vi "Open.vi"(7 "Allow multiple opens?":bool, 8 "error in (no error)":errorcluster, 10 "Channel Names":tag[](array[tag])) -> (0 "error out":errorcluster, 3 "AudioIn (N Samples) Ref Out":T1)   [LabVIEW 2021, in "AudioIn Block.lvlib"]
doc: "Opens a reference to audio input block read channels. You must open a reference before you read values from the audio input block read channels."
uses:
  <vilib>/myRIO/Instrument Drivers/Onboard IO/AudioIn Block/AudioIn Block.lvlib
  <vilib>/myRIO/Instrument Drivers/Onboard IO/AudioIn Block/typedefs/AudioIn Block Reference.ctl
  <vilib>/myRIO/Common/Instrument Driver Framework/Utilities/typedefs/myRIO Generic Hardware Reference.ctl
  <vilib>/myRIO/Common/Instrument Driver Framework/Utilities/typedefs/Hardware Version Enum.ctl
  <vilib>/myRIO/Common/Instrument Driver Framework/Utilities/typedefs/myRIO v1.0 Reference.ctl
  <vilib>/myRIO/Common/Instrument Driver Framework/Utilities/typedefs/Generic FPGA Reference.ctl
  <vilib>/myRIO/Common/Instrument Driver Framework/myRIO v1.0/AudioIn Block/typedefs/AudioIn Block Channels List.ctl
  <vilib>/myRIO/Common/Instrument Driver Framework/myRIO v1.0/AudioIn Block/typedefs/AudioIn Block Channels Enum.ctl
  <vilib>/myRIO/Common/Instrument Driver Framework/Utilities/typedefs/Analog Scaling Constants.ctl
  <vilib>/userdefined/High Color/nirio_resource_hc.ctl
panel:
  # "AudioIn (N Samples) Open"
  # "Opens a reference to the myRIO hardware and configures the AudioIn (N Samples) Reference with channels to be read"
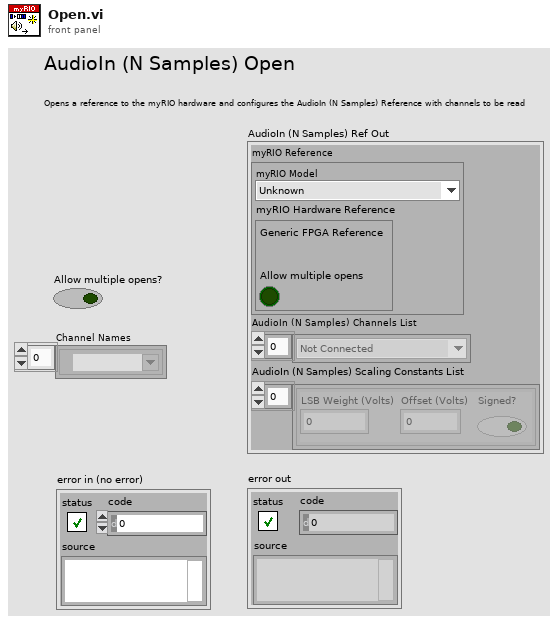
[diagram p1: front panel]
types:
  T1 = typedef "AudioIn Block.lvlib/AudioIn Block Reference.ctl" = cluster{"myRIO Reference":T2, "AudioIn (N Samples) Channels List":T6, "AudioIn (N Samples) Scaling Constants List":T8[]}
  T2 = typedef "myRIO Generic Hardware Reference.ctl" = cluster{"myRIO Model":T3, "myRIO Hardware Reference":T4}
  T3 = typedef "Hardware Version Enum.ctl" = enum16{"Unknown", "myRIO-1900", "myRIO-1950", "roboRIO", "NI ELVIS RIO CM", "ELVIS III"}
  T4 = typedef "myRIO v1.0 Reference.ctl" = cluster{"Generic FPGA Reference":T5, "Allow multiple opens":bool}
  T5 = typedef "Generic FPGA Reference.ctl" = refnum<k20>
  T6 = typedef "AudioIn Block Channels List.ctl" = T7[]
  T7 = typedef "AudioIn Block Channels Enum.ctl" = enum16{"Not Connected", "AudioIn/Left (N Samples)", "AudioIn/Right (N Samples)"}
  T8 = typedef "Analog Scaling Constants.ctl" = cluster{"LSB Weight (Volts)":dbl, "Offset (Volts)":dbl, "Signed?":bool}
  T9 = typedef "nirio_resource_hc.ctl" = tag
  T10 = typedef "Analog Scaling Constants List.ctl" = T8[]
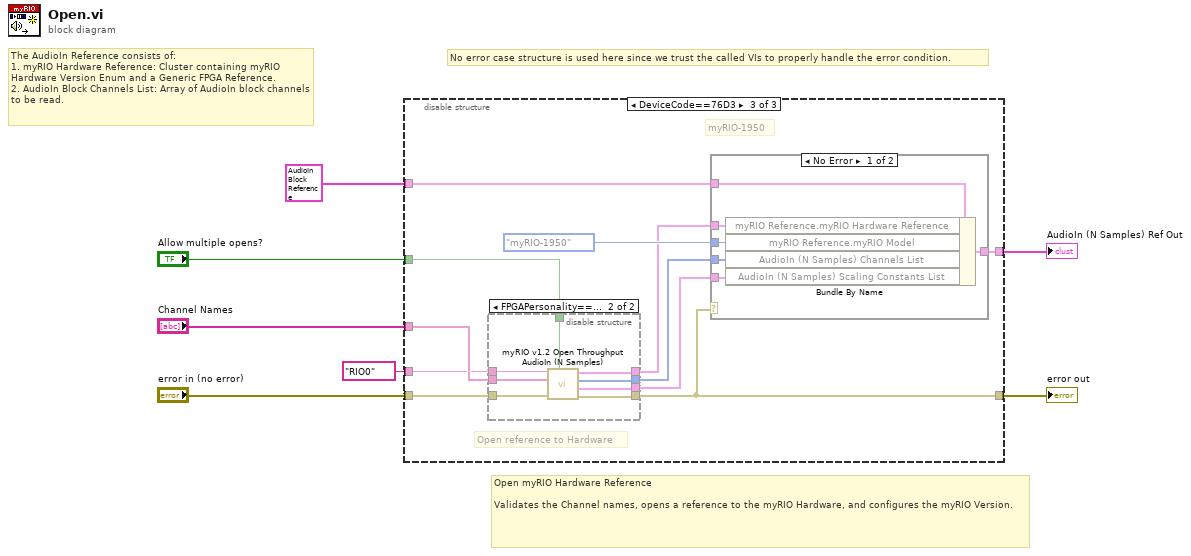
[diagram p0: block diagram]
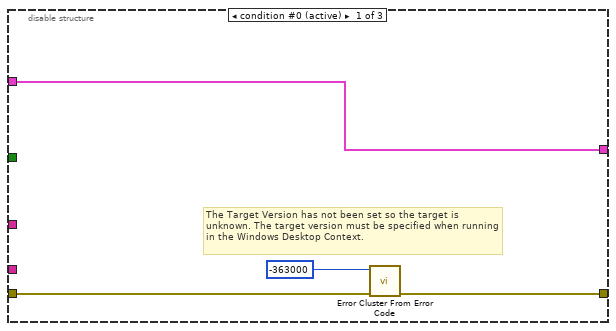
[diagram p2: hidden frame]
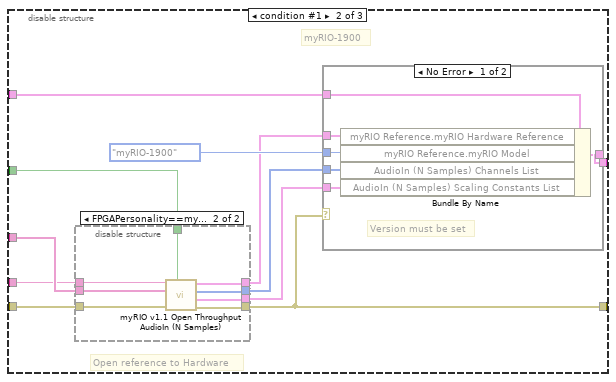
[diagram p3: hidden frame]
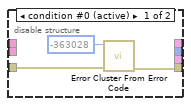
[diagram p4: hidden frame]
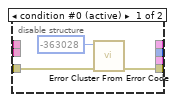
[diagram p6: hidden frame]
diagram:
  # "No error case structure is used here since we trust the called VIs to properly handle the error condition."
  # "The AudioIn Reference consists of:\n1. myRIO Hardware Reference: Cluster containing myRIO Hardware Version Enum and a Generic FPGA Reference.\n2. AudioIn Block Channels List: Array of AudioIn block channels to be read."
  # "Open myRIO Hardware Reference\n\nValidates the Channel names, opens a reference to the myRIO Hardware, and configures the myRIO Version."
  n1 = disable-structure shown="DeviceCode==76D3" {
    disable-tunnel: [w11 w14 w43] -> w4
    disable-tunnel: "Channel Names" -> [_ w22 w51]
    disable-tunnel: "Allow multiple opens?" -> [_ w18 w50]
    disable-tunnel: [w8 w21 w49] -> w1
    disable-tunnel: "error in (no error)" -> [w10 w19 w47]
    disable-tunnel: T1 {"myRIO Reference"={"myRIO Model"=enum."Unknown", "myRIO Hardware Reference"={"Generic FPGA Reference"=refnum, "Allow multiple opens"=FALSE}}, "AudioIn (N Samples) Channels List"=[], "AudioIn (N Samples) Scaling Constants List"=[]} ("AudioIn Block Read Ref Out") -> [w8 w17 w45]
    disable-tunnel: T9 "RIO0" ("Resource name") -> [_ w15 w44]
    frame condition #0 (active) {
      # "The Target Version has not been set so the target is unknown. The target version must be specified when running in the Windows Desktop Context."
      n2 = call <vilib>:"Error Cluster From Error Code.vi"("error in (no error)"=w10, "error code (0)"=-363000) -> ("error out"=w11:errorcluster)  [unwired: 7 in]
    }
    frame condition #1 {
      # "myRIO-1900"
      # "Open reference to Hardware"
      n3 = disable-structure shown="FPGAPersonality==myRIO_FP_Throughput" {
        disable-tunnel: w22 -> [_ w31]
        disable-tunnel: w19 -> [w24 w30]
        disable-tunnel: w18 -> [_ w33]
        disable-tunnel: [_ w28] -> w16
        disable-tunnel: w15 -> [_ w32]
        disable-tunnel: [w23 w26] -> w14
        disable-tunnel: [_ w29] -> w13
        disable-tunnel: [_ w27] -> w12
        frame condition #0 (active) {
          n4 = call <vilib>:"Error Cluster From Error Code.vi"("error in (no error)"=w24, "error code (0)"=-363028) -> ("error out"=w23:errorcluster)  [unwired: 7 in]
        }
        frame condition #1 {
          n5 = call <vilib>:"myRIO v1.1 Open Throughput AudioIn (N Samples).vi"("Allow multiple opens?"=w33, "error in (no error)"=w30, "Channel Names"=w31, "Resource name"=w32) -> ("error out"=w26:errorcluster, "AudioIn (N Samples) Scale Constants List"=w27:T10, "AudioIn (N Samples) Channel List"=w28:T6, "myRIO Ref Out"=w29:T4)  [unwired: 4 in]
        }
      }
      n6 = case shown="No Error" w14 {
        tunnel: [w39 w40] -> w21
        tunnel: Hardware_Version_Enum."myRIO-1900" ("Hardware Version Enum") -> [w38 _]
        tunnel: w17 -> [w37 w40]
        tunnel: w16 -> [w35 _]
        tunnel: w13 -> [w36 _]
        tunnel: w12 -> [w34 _]
        frame No Error {
          # "Version must be set"
          n7 = Bundle By Name(cluster=w37, "myRIO Reference.myRIO Hardware Reference"=w36, "myRIO Reference.myRIO Model"=w38, "AudioIn (N Samples) Channels List"=w35, "AudioIn (N Samples) Scaling Constants List"=w34) -> (w39:T1)
        }
        frame Error {
        }
      }
    }
    frame condition #2 {
      # "myRIO-1950"
      # "Open reference to Hardware"
      n8 = disable-structure shown="FPGAPersonality==myRIO_FP_Throughput" {
        disable-tunnel: w51 -> [_ w60]
        disable-tunnel: w50 -> [_ w62]
        disable-tunnel: w47 -> [w53 w59]
        disable-tunnel: [_ w58] -> w46
        disable-tunnel: w44 -> [_ w61]
        disable-tunnel: [w52 w55] -> w43
        disable-tunnel: [_ w57] -> w42
        disable-tunnel: [_ w56] -> w41
        frame condition #0 (active) {
          n9 = call <vilib>:"Error Cluster From Error Code.vi"("error in (no error)"=w53, "error code (0)"=-363028) -> ("error out"=w52:errorcluster)  [unwired: 7 in]
        }
        frame condition #1 {
          n10 = call <vilib>:"myRIO v1.2 Open Throughput AudioIn (N Samples).vi"("Allow multiple opens?"=w62, "error in (no error)"=w59, "Channel Names"=w60, "Resource name"=w61) -> ("error out"=w55:errorcluster, "AudioIn (N Samples) Scale Constants List"=w56:T10, "AudioIn (N Samples) Channel List"=w57:T6, "myRIO Ref Out"=w58:T4)  [unwired: 4 in]
        }
      }
      n11 = case shown="No Error" w43 {
        tunnel: [w68 w69] -> w49
        tunnel: Hardware_Version_Enum."myRIO-1950" ("Hardware Version Enum") -> [w67 _]
        tunnel: w46 -> [w64 _]
        tunnel: w45 -> [w66 w69]
        tunnel: w42 -> [w65 _]
        tunnel: w41 -> [w63 _]
        frame No Error {
          n12 = Bundle By Name(cluster=w66, "myRIO Reference.myRIO Hardware Reference"=w64, "myRIO Reference.myRIO Model"=w67, "AudioIn (N Samples) Channels List"=w65, "AudioIn (N Samples) Scaling Constants List"=w63) -> (w68:T1)
        }
        frame Error {
        }
      }
    }
  }
  "AudioIn (N Samples) Ref Out" <- w1
  "error out" <- w4
